vi "Teleop.vi"(10 "Match Info":T2={"Autonomous Elapsed Seconds"=0.0, "TeleOp Elapsed Seconds"=0.0, "Disabled Elapsed Seconds"=0.0, "Visited Autonomous"=FALSE, "Visited TeleOp"=FALSE, "Visited Disabled"=FALSE, "Autonomous Settings"={"Autonomous Style"=enum."Independent", "VI Refnum"=refnum}}, 11 "Call Context":T3) -> ()   [LabVIEW 2016]
doc: "This VI is called for each TeleOp packet received from the DS where the robot is not disabled. It is often used to read from the joysticks and update I/O or to update setpoints for timed control loops. It should complete and return within 20 milliseconds or it may miss DS packets."
uses:
  <vilib>/Rock Robotics/WPI/DriverStation/WPI_DriverStationDerivedRobotMode.ctl
  <vilib>/Rock Robotics/WPI/DriverStation/WPI_DriverStationMatch Info.ctl
  <userlib>/836-libraries/Drive/Drive_Code/Drive_Code_Support/Drive_Code_PID_Bundle.ctl
  FMS Commands.ctl
  Drive Commands.ctl
  <userlib>/836-libraries/Drive/Drive_Code/Drive_Code_Support/Sensor_Cluster.ctl
  <userlib>/836-libraries/Drive/Drive_Code/Drive_Code_Support/Camera_Cluster.ctl
  <userlib>/836-libraries/Drive/Drive_Code/Drive_Code_Support/Drive_Code_Notifier.ctl
  <userlib>/836-libraries/Drive/Drive_Code/Drive_Code_Support/Drive_Code_Command.ctl
  <userlib>/836-libraries/Drive/Drive_Code/Logging_Data.ctl
  <vilib>/Rock Robotics/WPI/Utilities/WPI_GetSetVariantRefNum.vi
panel:
  in  "Tab Control":enum32{"Drive", "Page 2"}(tab)
  in  "High Gear PID":T1={"Yaw, Driving Straight"={"proportional gain (Kc)"=1.0, "integral time (Ti, min)"=0.01, "derivative time (Td, min)"=0.0}, "Yaw, Holding Still"={"proportional gain (Kc)"=1.0, "integral time (Ti, min)"=0.01, "derivative time (Td, min)"=0.0}, "Distance, Driving Straight"={"proportional gain (Kc)"=1.0, "integral time (Ti, min)"=0.01, "derivative time (Td, min)"=0.0}, "Distance, Holding Still"={"proportional gain (Kc)"=1.0, "integral time (Ti, min)"=0.01, "derivative time (Td, min)"=0.0}}
  in  "Low Gear PID":T1={"Yaw, Driving Straight"={"proportional gain (Kc)"=1.0, "integral time (Ti, min)"=0.01, "derivative time (Td, min)"=0.0}, "Yaw, Holding Still"={"proportional gain (Kc)"=1.0, "integral time (Ti, min)"=0.01, "derivative time (Td, min)"=0.0}, "Distance, Driving Straight"={"proportional gain (Kc)"=1.0, "integral time (Ti, min)"=0.01, "derivative time (Td, min)"=0.0}, "Distance, Holding Still"={"proportional gain (Kc)"=1.0, "integral time (Ti, min)"=0.01, "derivative time (Td, min)"=0.0}}
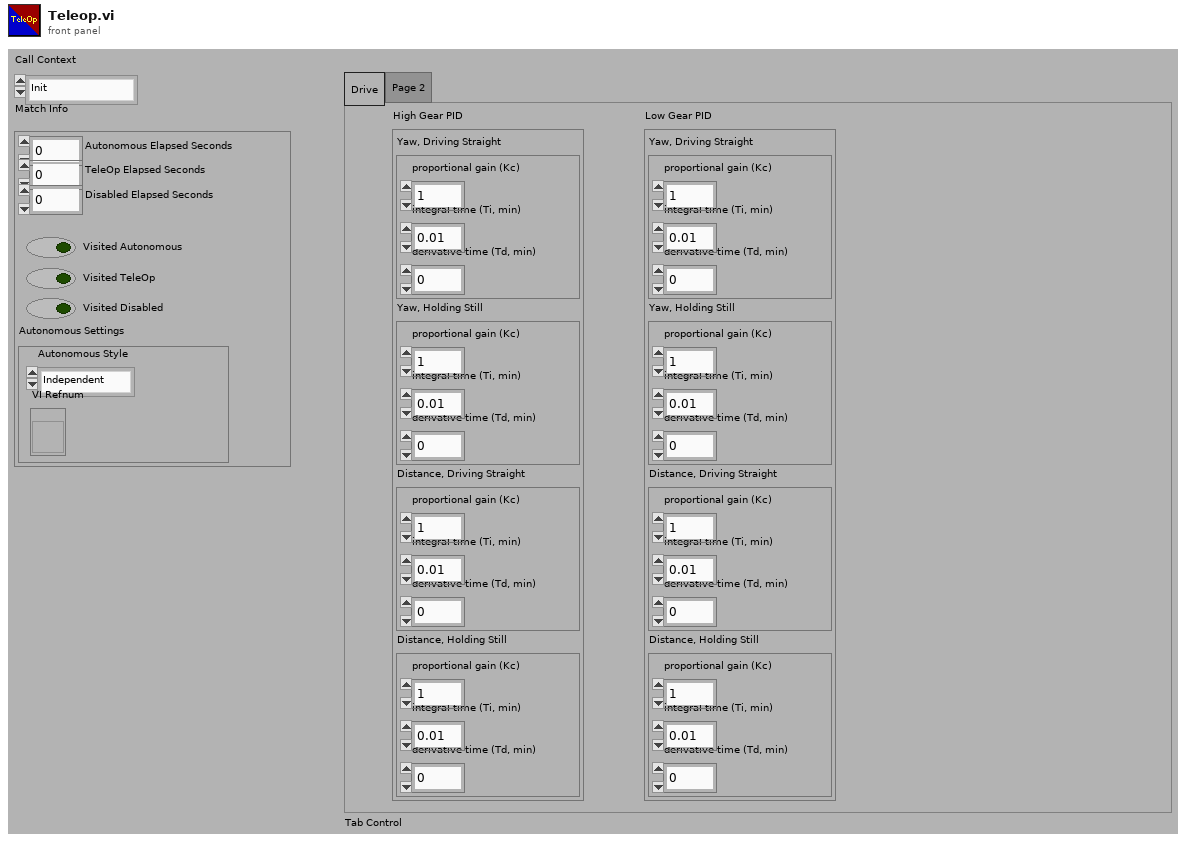
[diagram p1: front panel]
types:
  T1 = typedef "Drive_Code_PID_Bundle.ctl" = cluster{"Yaw, Driving Straight":cluster{"proportional gain (Kc)":dbl, "integral time (Ti, min)":dbl, "derivative time (Td, min)":dbl}, "Yaw, Holding Still":cluster{"proportional gain (Kc)":dbl, "integral time (Ti, min)":dbl, "derivative time (Td, min)":dbl}, "Distance, Driving Straight":cluster{"proportional gain (Kc)":dbl, "integral time (Ti, min)":dbl, "derivative time (Td, min)":dbl}, "Distance, Holding Still":cluster{"proportional gain (Kc)":dbl, "integral time (Ti, min)":dbl, "derivative time (Td, min)":dbl}}
  T2 = typedef "WPI_DriverStationMatch Info.ctl" = cluster{"Autonomous Elapsed Seconds":dbl, "TeleOp Elapsed Seconds":dbl, "Disabled Elapsed Seconds":dbl, "Visited Autonomous":bool, "Visited TeleOp":bool, "Visited Disabled":bool, "Autonomous Settings":cluster{"Autonomous Style":enum16{"Iterative", "Independent"}, "VI Refnum":refnum<vi>}}
  T3 = typedef "WPI_DriverStationDerivedRobotMode.ctl" = enum16{"Init", "Execute", "Stop"}
  T4 = typedef "WPI_JoystickDevRef.ctl" = cluster{"Device":T5}
  T5 = typedef "WPI_JoystickDeviceEnum.ctl" = enum16{"USB 0", "USB 1", "USB 2", "USB 3", "USB 4", "USB 5"}
  T6 = typedef "FMS Commands.ctl" = enum16{"Shoot", "Un-Jam", "Stop"}
  T7 = typedef "Drive Commands.ctl" = enum16{"Manual", "Get Gear", "Score Gear", "Align Rope"}
  T8 = typedef "Sensor_Cluster.ctl" = cluster{"Gyro Data":cluster{"Gyro RT FIFO":refnum<k33>, "Gyro Current":dbl, "Gyro Hold":dbl}, "Encoder Data":cluster{"Encoder RT FIFO":refnum<k33>, "Encoder Current":dbl, "Encoder Hold":dbl}, "Camera Data":cluster{"Camera RT FIFO":refnum<k33>, "Camera Current":T9}}
  T9 = typedef "Camera_Cluster.ctl" = cluster{" Angle":dbl, "Valid":bool}
  T10 = cluster{"Cluster":T8, "Drive Command rt fifo":refnum<k33>, "Logging Data":refnum<k33>, "PID Update":refnum<notifier>}
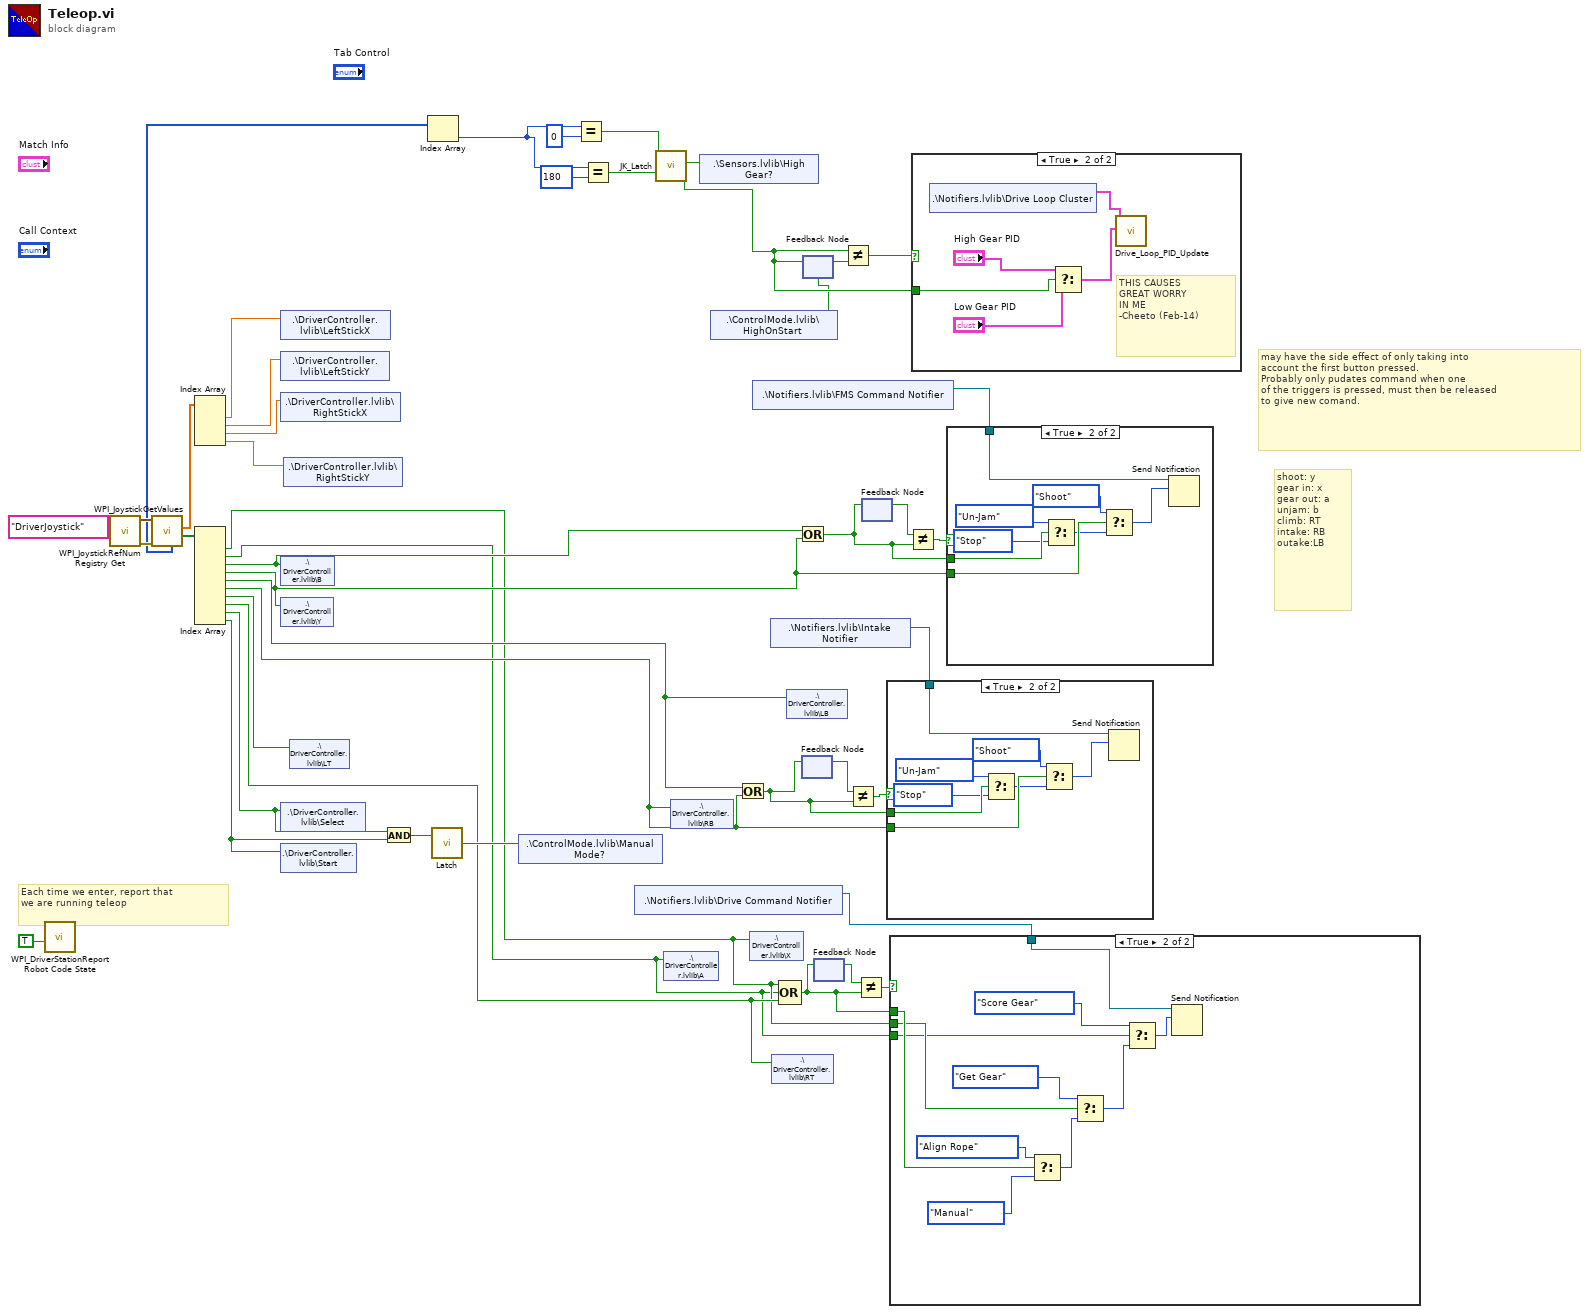
[diagram p0: block diagram]
diagram:
  # "shoot: y\ngear in: x\ngear out: a\nunjam: b\nclimb: RT\nintake: RB\noutake:LB"
  # "may have the side effect of only taking into\naccount the first button pressed.\nProbably only pudates command when one\nof the triggers is pressed, must then be released\nto give new comand."
  # "Each time we enter, report that\nwe are running teleop"
  n1 = call <vilib>:"WPI_DriverStationReport Robot Code State.vi"("TeleOp"=TRUE ("Autonomous")) -> ()  [unwired: 10 in, 1 out]
  n2 = call <vilib>:"WPI_JoystickRefNum Registry Get.vi"("refnum name"="DriverJoystick") -> ("error out"=w42:errorcluster, "JoystickDevRef"=w41:T4)  [unwired: 9 in]
  n3 = call <vilib>:"WPI_JoystickGetValues.vi"("error in (no error)"=w42, "JoystickDevRef"=w41) -> ("Buttons"=w39:bool[], "Axes"=w40:dbl[], "POVs"=w33:i16[])  [unwired: 5 in, 2 out]
  n4 = Index Array(array=w40) -> (element #1=w38:dbl, element #2=w36:dbl, element #3=w10:dbl, element #4=w37:dbl)  [unwired: 4 in]
  n5 = Index Array(array=w39) -> (element #1=w4:bool, element #2=w2:bool, element #3=w14:bool, element #4=w15:bool, element #5=w12:bool, element #6=w13:bool, element #7=w9:bool, element #8=w8:bool, element #9=w23:bool, element #10=w22:bool)  [unwired: 10 in]
  n6 = shared-variable ".\\DriverController.lvlib\\LeftStickX"(w38) -> ()  [unwired: 1 in, 1 out]
  n7 = shared-variable ".\\DriverController.lvlib\\LeftStickY"(w36) -> ()  [unwired: 1 in, 1 out]
  n8 = shared-variable ".\\DriverController.lvlib\\RightStickX"(w10) -> ()  [unwired: 1 in, 1 out]
  n9 = shared-variable ".\\DriverController.lvlib\\B"(w14) -> ()  [unwired: 1 in, 1 out]
  n10 = shared-variable ".\\DriverController.lvlib\\Y"(w15) -> ()  [unwired: 1 in, 1 out]
  n11 = shared-variable ".\\DriverController.lvlib\\Select"(w23) -> ()  [unwired: 1 in, 1 out]
  n12 = shared-variable ".\\DriverController.lvlib\\Start"(w22) -> ()  [unwired: 1 in, 1 out]
  n13 = shared-variable ".\\DriverController.lvlib\\RightStickY"(w37) -> ()  [unwired: 1 in, 1 out]
  n14 = shared-variable ".\\DriverController.lvlib\\LT"(w9) -> ()  [unwired: 1 in, 1 out]
  n15 = And(x=w23, y=w22) -> (x .and. y?=w21:bool)
  n16 = Index Array(array=w33) -> (element=w30:i16)  [unwired: 1 in]
  n17 = call <userlib>:"Latch.vi"("In"=w21) -> ("Out"=w20:bool)  [unwired: 1 in]
  n18 = shared-variable ".\\ControlMode.lvlib\\Manual Mode?"(w20) -> ()  [unwired: 1 in, 1 out]
  n19 = Equal?(x=w30, y=i16 0) -> (x = y?=w29:bool)
  n20 = Equal?(x=w30, y=i16 180) -> (x = y?=w28:bool)
  n21 = shared-variable ".\\Notifiers.lvlib\\Drive Command Notifier"() -> (w5:refnum<notifier>)  [unwired: 1 in, 1 out]
  n22 = call <userlib>:"JK_Latch.vi"("Reset"=w28, "Set"=w29) -> ("Q"=w27:bool)  [unwired: 5 in]
  n23 = shared-variable ".\\DriverController.lvlib\\A"(w2) -> ()  [unwired: 1 in, 1 out]
  n24 = shared-variable ".\\DriverController.lvlib\\RB"(w13) -> ()  [unwired: 1 in, 1 out]
  n25 = shared-variable ".\\Sensors.lvlib\\High Gear?"(w27) -> ()  [unwired: 1 in, 1 out]
  n26 = shared-variable ".\\ControlMode.lvlib\\HighOnStart"() -> (w1:bool)  [unwired: 1 in, 1 out]
  n27 = Or(x=w12, y=w13) -> (x .or. y?=w18:bool)
  n28 = shared-variable ".\\DriverController.lvlib\\X"(w4) -> ()  [unwired: 1 in, 1 out]
  n29 = shared-variable ".\\Notifiers.lvlib\\FMS Command Notifier"() -> (w19:refnum<notifier>)  [unwired: 1 in, 1 out]
  n30 = shared-variable ".\\Notifiers.lvlib\\Intake Notifier"() -> (w11:refnum<notifier>)  [unwired: 1 in, 1 out]
  n31 = shared-variable ".\\DriverController.lvlib\\RT"(w8) -> ()  [unwired: 1 in, 1 out]
  n32 = Compound Arithmetic op=OR(w4, w2, w8) -> (w3:bool)
  n33 = shared-variable ".\\DriverController.lvlib\\LB"(w12) -> ()  [unwired: 1 in, 1 out]
  n34 = Or(x=w14, y=w15) -> (x .or. y?=w24:bool)
  n35 = feedback #1() -> (w16:bool)  [unwired: 1 in]
  n36 = feedback-in #1(w18) -> ()
  n37 = feedback-in #2(w27) -> ()
  n38 = feedback #2(w1) -> (w35:bool)
  n39 = feedback-in #3(w3) -> ()
  n40 = feedback #3() -> (w6:bool)  [unwired: 1 in]
  n41 = Not Equal?(x=w27, y=w35) -> (x != y?=w34:bool)
  n42 = Not Equal?(x=w16, y=w18) -> (x != y?=w17:bool)
  n43 = Not Equal?(x=w6, y=w3) -> (x != y?=w7:bool)
  n44 = feedback-in #4(w24) -> ()
  n45 = feedback #4() -> (w26:bool)  [unwired: 1 in]
  n46 = case shown="True" w17 {
    tunnel: w11 -> [_ w52]
    tunnel: w18 -> [_ w51]
    tunnel: w13 -> [_ w50]
    frame False {
    }
    frame True {
      n47 = Select(t=FMS_Commands."Un-Jam" ("Enum"), s=w51, f=FMS_Commands."Stop" ("Enum")) -> (s? t:f=w48:T6)
      n48 = Select(t=FMS_Commands."Shoot" ("Enum"), s=w50, f=w48) -> (s? t:f=w45:T6)
      n49 = Send Notification(notification=w45, notifier=w52) -> ()  [unwired: 1 in, 2 out]
    }
  }
  n50 = case shown="True" w7 {
    tunnel: w5 -> [_ w63]
    tunnel: w4 -> [_ w61]
    tunnel: w3 -> [_ w62]
    tunnel: w2 -> [_ w60]
    frame False {
    }
    frame True {
      n51 = Select(t=Drive_Commands."Align Rope" ("Enum"), s=w62, f=Drive_Commands."Manual" ("Enum")) -> (s? t:f=w55:T7)
      n52 = Select(t=Drive_Commands."Get Gear" ("Enum"), s=w61, f=w55) -> (s? t:f=w54:T7)
      n53 = Select(t=Drive_Commands."Score Gear" ("Enum"), s=w60, f=w54) -> (s? t:f=w53:T7)
      n54 = Send Notification(notification=w53, notifier=w63) -> ()  [unwired: 1 in, 2 out]
    }
  }
  n55 = Not Equal?(x=w26, y=w24) -> (x != y?=w25:bool)
  n56 = case shown="True" w34 {
    tunnel: w27 -> [_ w68]
    frame False {
    }
    frame True {
      # "THIS CAUSES\nGREAT WORRY\nIN ME\n-Cheeto (Feb-14)"
      n57 = shared-variable ".\\Notifiers.lvlib\\Drive Loop Cluster"() -> (w64:T10)  [unwired: 1 in, 1 out]
      n58 = Select(t="High Gear PID", s=w68, f="Low Gear PID") -> (s? t:f=w65:T1)
      n59 = call <userlib>:"Drive_Loop_PID_Update.vi"("PID Gains"=w65, "Control Cluster"=w64) -> ()  [unwired: 10 in]
    }
  }
  n60 = case shown="True" w25 {
    tunnel: w19 -> [_ w76]
    tunnel: w24 -> [_ w75]
    tunnel: w15 -> [_ w74]
    frame False {
    }
    frame True {
      n61 = Select(t=FMS_Commands."Un-Jam" ("Enum"), s=w75, f=FMS_Commands."Stop" ("Enum")) -> (s? t:f=w72:T6)
      n62 = Select(t=FMS_Commands."Shoot" ("Enum"), s=w74, f=w72) -> (s? t:f=w69:T6)
      n63 = Send Notification(notification=w69, notifier=w76) -> ()  [unwired: 1 in, 2 out]
    }
  }
